vi "DataStore.vi"(7 "operation":T4=enum."GetWfms", 8 "error in (no error)":errorcluster, 9 "data in":T1, 11 "group":string) -> (0 "error out":errorcluster, 1 "data out":T1)   [LabVIEW 2017, in "DataAccumulator.lvlib"]
uses:
  <vilib>/addons/InsightCM/Devices/Shared/Common/DataAccumulator/DataAccumulator.lvlib
  <vilib>/addons/InsightCM/Devices/Shared/Common/DataAccumulator/controls/DataStoreOps.ctl
  <vilib>/addons/InsightCM/Devices/Shared/Common/DataAccumulator/controls/DataStoreType.ctl
  <vilib>/addons/InsightCM/Utilities/Analysis/Shared/controls/PulsePositions.ctl
  <vilib>/addons/InsightCM/Devices/Shared/Common/DVRBuffer/controls/BufferLocation.ctl
  <vilib>/addons/InsightCM/Utilities/Analysis/Shared/AnalysisHelper.lvlib
  <vilib>/addons/InsightCM/Devices/Shared/Common/DVRBuffer/DVRBuffer.lvlib
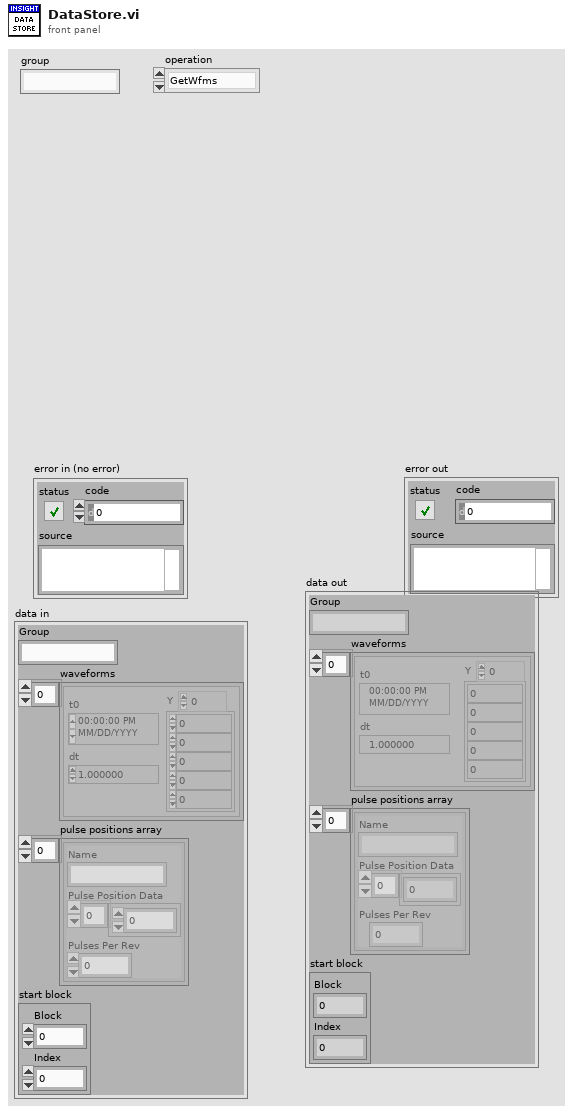
[diagram p1: front panel]
types:
  T1 = typedef "DataAccumulator.lvlib/DataStoreType.ctl" = cluster{"Group":string, "waveforms":waveform(sgl)[], "pulse positions array":T2[], "start block":T3}
  T2 = typedef "AnalysisHelper.lvlib/PulsePositions.ctl" = cluster{"Name":string, "Pulse Position Data":dbl[], "Pulses Per Rev":i32}
  T3 = typedef "DVRBuffer.lvlib/BufferLocation.ctl" = cluster{"Block":u32, "Index":i32}
  T4 = typedef "DataAccumulator.lvlib/DataStoreOps.ctl" = enum16{"Reset", "Init", "Clear", "SetWfms", "GetWfms"}
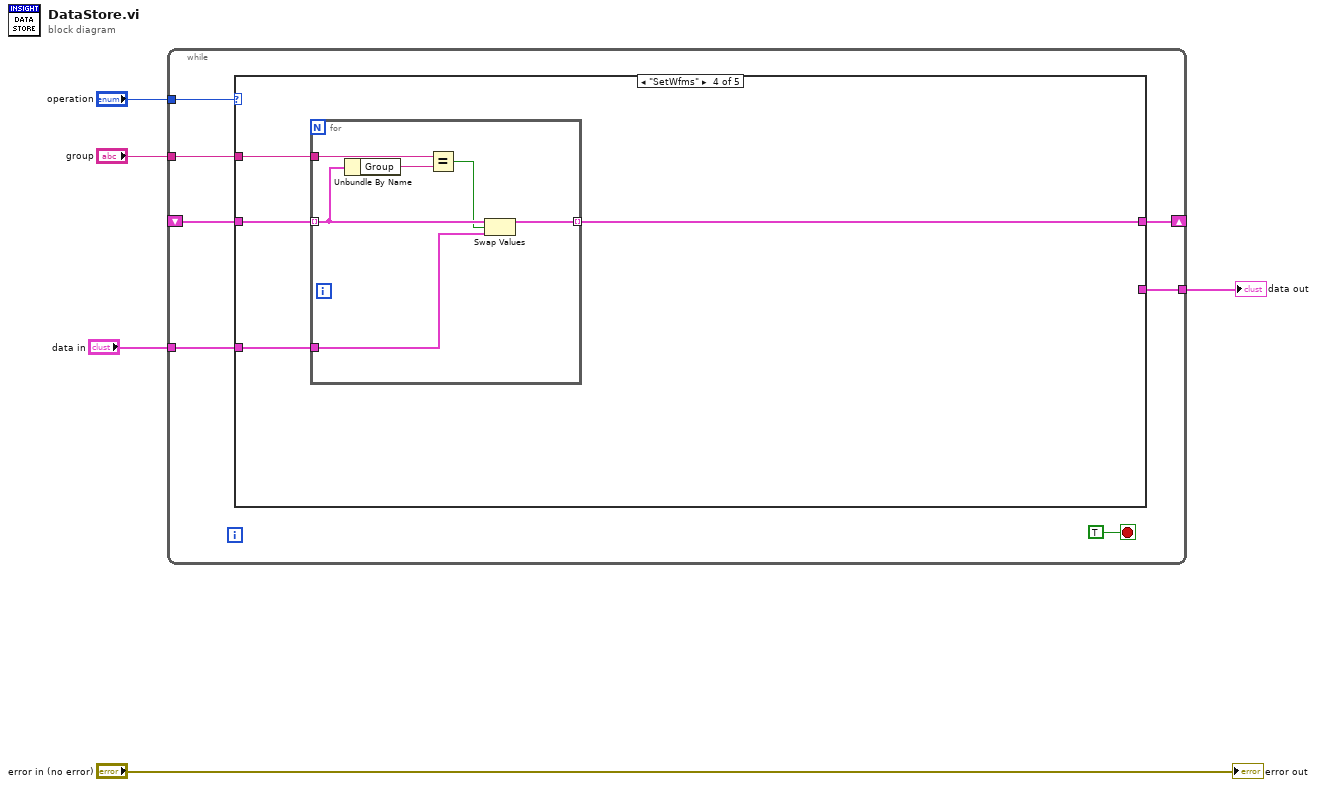
[diagram p0: block diagram]
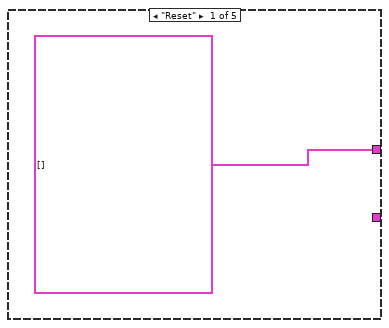
[diagram p2: hidden frame]
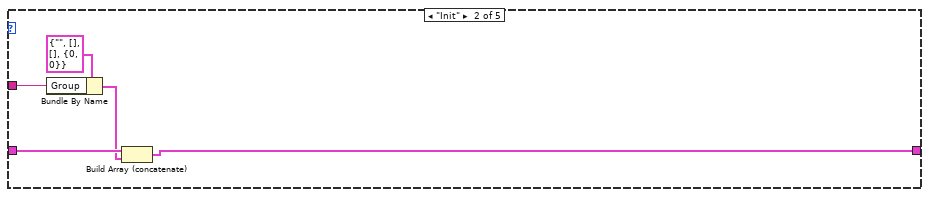
[diagram p3: hidden frame]
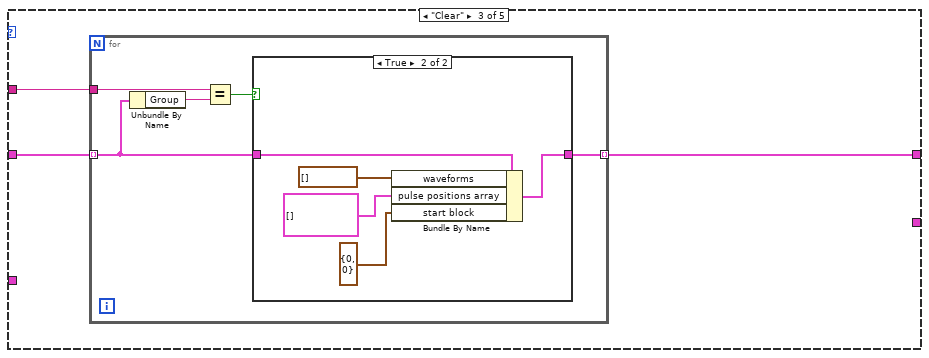
[diagram p4: hidden frame]
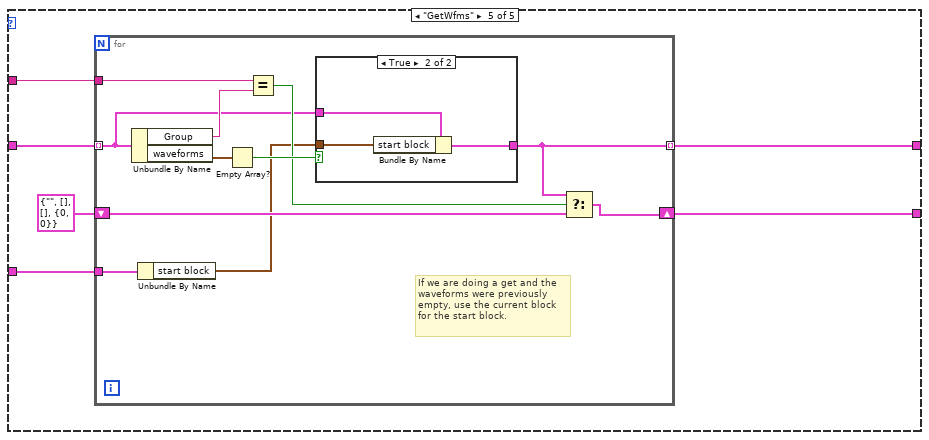
[diagram p6: hidden frame]
diagram:
  n1 = while {
    tunnel: "operation" -> [w11]
    tunnel: "group" -> [w10]
    tunnel: "data in" -> [w9]
    tunnel: [w8] -> w1
    shift-right: [w7] -> _
    shift-left: _ -> [w6]
    stop <- TRUE stop-if-true
    n2 = case shown="\"SetWfms\"" w11 {
      tunnel: w10 -> [_ w17 w20 w35 w48]
      tunnel: w9 -> [_ _ _ w34 w43]
      tunnel: [_ _ _ _ w44] -> w8
      tunnel: [T1[] [] w14 w19 w33 w45] -> w7
      tunnel: w6 -> [_ w16 w21 w36 w47]
      frame "Reset" {
      }
      frame "Init" {
        n3 = Bundle By Name(cluster=T1 {"Group"="", "waveforms"=[], "pulse positions array"=[], "start block"={"Block"=0, "Index"=0}} ("DataStoreType"), "Group"=w17) -> (w15:T1)
        n4 = Build Array (concatenate)(w16, w15) -> (w14:T1[])
      }
      frame "Clear" {
        n5 = for {
          tunnel: w21 -> [w23] mode=indexing
          tunnel: w20 -> [w25]
          tunnel: [w22] -> w19 mode=indexing
          n6 = Unbundle By Name(w23) -> ("Group"=w26:string)
          n7 = Equal?(x=w25, y=w26) -> (x = y?=w24:bool)
          n8 = case shown="True" w24 {
            tunnel: w23 -> [w27 w32]
            tunnel: [w27 w31] -> w22
            frame False {
            }
            frame True {
              n9 = Bundle By Name(cluster=w32, "waveforms"=waveform(sgl)[] [], "pulse positions array"=T2[] [], "start block"=T3 {"Block"=0, "Index"=0}) -> (w31:T1)
            }
          }
        }
      }
      frame "SetWfms" {
        n10 = for {
          tunnel: w36 -> [w38] mode=indexing
          tunnel: w35 -> [w41]
          tunnel: w34 -> [w40]
          tunnel: [w39] -> w33 mode=indexing
          n11 = Unbundle By Name(w38) -> ("Group"=w42:string)
          n12 = Equal?(x=w41, y=w42) -> (x = y?=w37:bool)
          n13 = Swap Values(12:w38, 13:w37, 14:w40) -> (1:w39:T1)  [unwired: 1 out]
        }
      }
      frame "GetWfms" {
        n14 = for {
          tunnel: w48 -> [w58]
          tunnel: w47 -> [w54] mode=indexing
          shift-right: [w52] -> w44
          shift-left: T1 {"Group"="", "waveforms"=[], "pulse positions array"=[], "start block"={"Block"=0, "Index"=0}} ("DataStoreType") -> [w53]
          tunnel: [w49] -> w45 mode=indexing
          tunnel: w43 -> [w51]
          # "If we are doing a get and the\nwaveforms were previously\nempty, use the current block\nfor the start block."
          n15 = Unbundle By Name(w54) -> ("Group"=w59:string, "waveforms"=w57:waveform(sgl)[])
          n16 = Unbundle By Name(w51) -> ("start block"=w50:T3)
          n17 = Empty Array?(array=w57) -> (empty?=w56:bool)
          n18 = Equal?(x=w58, y=w59) -> (x = y?=w55:bool)
          n19 = case shown="True" w56 {
            tunnel: w50 -> [_ w61]
            tunnel: w54 -> [w60 w63]
            tunnel: [w60 w62] -> w49
            frame False {
            }
            frame True {
              n20 = Bundle By Name(cluster=w63, "start block"=w61) -> (w62:T1)
            }
          }
          n21 = Select(t=w49, s=w55, f=w53) -> (s? t:f=w52:T1)
        }
      }
    }
  }
  "data out" <- w1
  "error out" <- "error in (no error)"
